vi "Measurement Logic.vi"(8 "error in":errorcluster, 9 "measurement configuration":T2 {"Baudrate" format="%x"; "FD Baudrate" format="%x"}, 10 "measure call context in":refnum<class "Measure Call Context.lvclass">) -> (0 "error out":errorcluster, 1 "measurement results":T1, 2 "measure call context out":refnum<class "Measure Call Context.lvclass">)   [LabVIEW 2025, in "CAN-LIN Raw Bus Capture.lvclass"]
doc: "Contains the core logic for executing the measurement."
uses:
  CAN-LIN Raw Bus Capture.lvclass
  <vilib>/Plug-In SDKs/Measurements/Measure Call Context/Measure Call Context.lvclass
  Measurement Configuration.ctl
  CAN-LIN Raw Bus Capture UI/Toggle.ctl
  Measurement Results.ctl
  <vilib>/xnet/xnet.llb/XNET Read (Frame CAN).vi
  CAN-LIN Raw Bus Capture.lvclass/CAN-LIN Raw Bus Capture.ctl
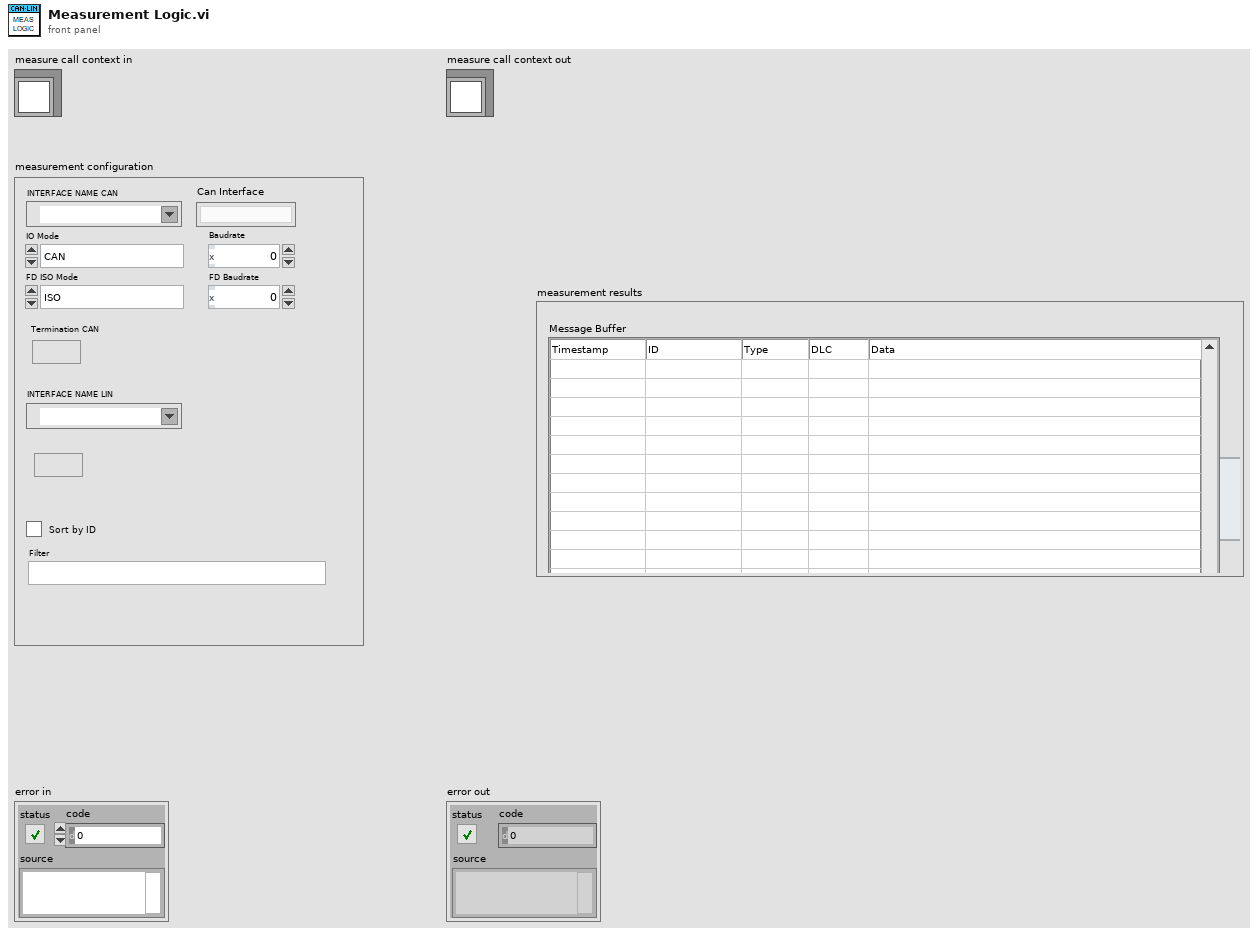
[diagram p1: front panel]
types:
  T1 = typedef "CAN-LIN Raw Bus Capture.lvclass/Measurement Results.ctl" = cluster{"CAN Bus Info":string, "Message Buffer":string[][]}
  T2 = typedef "CAN-LIN Raw Bus Capture.lvclass/Measurement Configuration.ctl" = cluster{"INTERFACE NAME CAN":refnum<k21>, "Termination CAN":T3, "FD Baudrate":u32, "Baudrate":u32, "FD ISO Mode":enum32{"ISO", "Legacy ISO", "Non-ISO"}, "IO Mode":enum32{"CAN", "CAN FD", "CAN FD + BRS"}, "SortByID":bool, "Filter":string, "INTERFACE NAME LIN":refnum<k21>, "Termination LIN":T3, "Can Interface":string}
  T3 = typedef "Toggle.ctl" = bool
  T4 = typedef "XNET Frame CAN.ctl" = cluster{"timestamp":timestamp, "payload":u8[], "identifier":u32, "type":T5, "extended?":bool, "echo?":bool}
  T5 = typedef "XNET Frame Type CAN.ctl" = u8
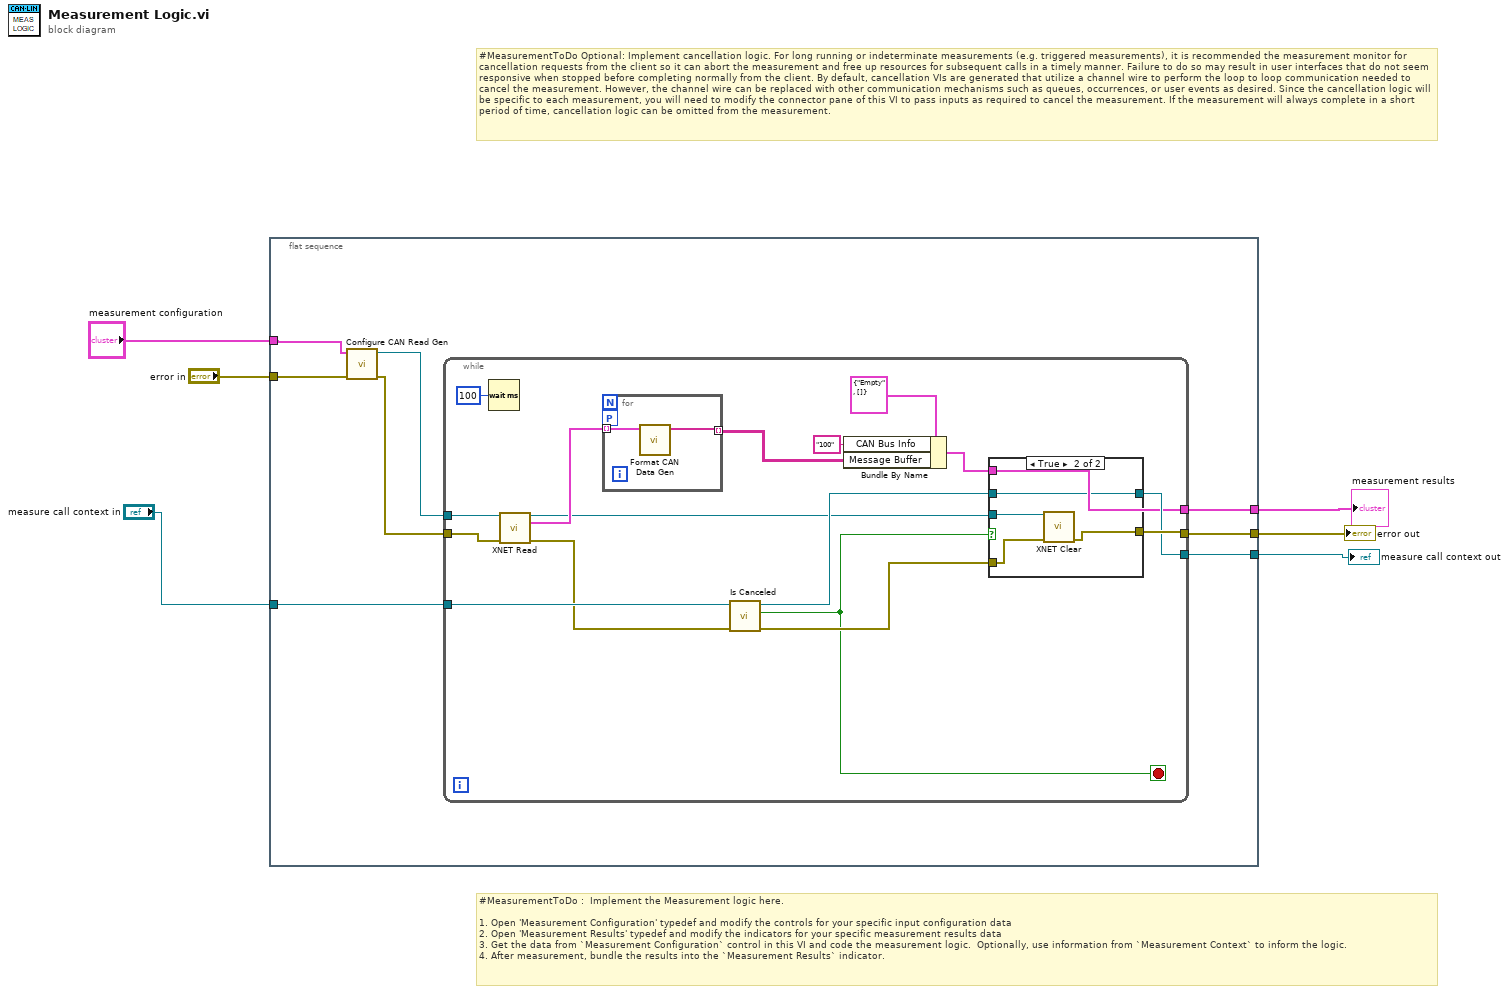
[diagram p0: block diagram]
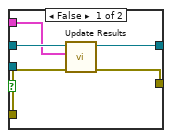
[diagram p2: hidden frame]
diagram:
  # "#MeasurementToDo Optional: Implement cancellation logic. For long running or indeterminate measurements (e.g. triggered measurements), it is recommended the measurement monitor for cancellation requests from the client so it can abort the measurement and free up resources for subsequent calls in a timely manner. Failure to do so may result in user interfaces that do not seem responsive when stopped before completing normally from the client. By default, cancellation VIs are generated that utilize a channel wire to perform the loop to loop communication needed to cancel the measurement. However, the channel wire can be replaced with other communication mechanisms such as queues, occurrences, or user events as desired. Since the cancellation logic will be specific to each measurement, you will need to modify the connector pane of this VI to pass inputs as required to cancel the measurement. If the measurement will always complete in a short period of time, cancellation logic can be omitted from the measurement."
  # "#MeasurementToDo :  Implement the Measurement logic here.\n\n1. Open 'Measurement Configuration' typedef and modify the controls for your specific input configuration data\n2. Open 'Measurement Results' typedef and modify the indicators for your specific measurement results data\n3. Get the data from `Measurement Configuration` control in this VI and code the measurement logic.  Optionally, use information from `Measurement Context` to inform the logic.\n4. After measurement, bundle the results into the `Measurement Results` indicator."
  n1 = flat-sequence {
    tunnel: "measurement configuration" -> [w10]
    tunnel: [w14] -> w4
    tunnel: "error in" -> [w7]
    tunnel: "measure call context in" -> [w13]
    tunnel: [w12] -> w2
    tunnel: [w11] -> w1
    frame #0 {
      n2 = call "Configure CAN Read Gen.vi"("error in"=w7, "measurement configuration"=w10) -> ("error out"=w8:errorcluster, "XNET Read"=w9:refnum<k21>)  [unwired: 8 in]
      n3 = while {
        tunnel: [w17] -> w14
        tunnel: w13 -> [w26]
        tunnel: w9 -> [w24]
        tunnel: [w19] -> w11
        tunnel: w8 -> [w25]
        tunnel: [w20] -> w12
        stop <- w16 stop-if-true
        n4 = Wait (ms)(milliseconds to wait=u32 100) -> ()  [unwired: 1 out]
        n5 = call-poly <vilib>:"XNET Read.vi"("session in"=w24, "error in (no error)"=w25) -> ("session out"=w18:refnum<k21>, "data"=w23:T4[], "error out"=w15:errorcluster)  [unwired: 10 in, 1 out]
        n6 = for {
          tunnel: w23 -> [w32] mode=indexing
          tunnel: [w31] -> w27 mode=indexing
          workers-P: _ -> [_]
          n7 = call "Format CAN Data Gen.vi"("Frame"=w32) -> ("Display"=w31:string[])  [unwired: 8 in, 2 out]
        }
        n8 = call <vilib>:"Is Canceled.vi"("error in"=w15, "measure call context in"=w26) -> ("error out"=w21:errorcluster, "is canceled?"=w16:bool, "measure call context out"=w22:refnum<class "Measure Call Context.lvclass">)  [unwired: 7 in]
        n9 = Bundle By Name(cluster=T1 {"CAN Bus Info"="Empty", "Message Buffer"=[]} ("Measurement Results"), "CAN Bus Info"="100", "Message Buffer"=w27) -> (w17:T1)
        n10 = case shown="True" w16 {
          tunnel: w22 -> [w37 w38]
          tunnel: w21 -> [w36 w41]
          tunnel: [w35 w40] -> w20
          tunnel: [w34 w38] -> w19
          tunnel: w18 -> [_ w39]
          tunnel: w17 -> [w33 _]
          frame False {
            n11 = call <vilib>:"Update Results.vi"("error in"=w36, "measurement results"=w33, "measure call context in"=w37) -> ("error out"=w35:errorcluster, "measure call context out"=w34:refnum<class "Measure Call Context.lvclass">)  [unwired: 7 in]
          }
          frame True {
            n12 = call <vilib>:"XNET Clear.vi"("session in"=w39, "error in (no error)"=w41) -> ("error out"=w40:errorcluster)  [unwired: 13 in]
          }
        }
      }
    }
  }
  "error out" <- w2
  "measure call context out" <- w1
  "measurement results" <- w4
